vi "tagDB_setValue_Template.vi"(8 "Error In":errorcluster, 9 "value":variant, 10 "name":string, 11 "DB Ref":T1) -> (0 "Error Out":errorcluster, 1 "created?":bool, 3 "DB Ref(dup)":T1)   [LabVIEW 2014, in "TagDB(dev).lvlib"]
doc: "[Covers: REQ_TAGDB_TEMPLATE_SETVALUE]"
uses:
  tagDB_Def.ctl
  TagDB(dev).lvlib
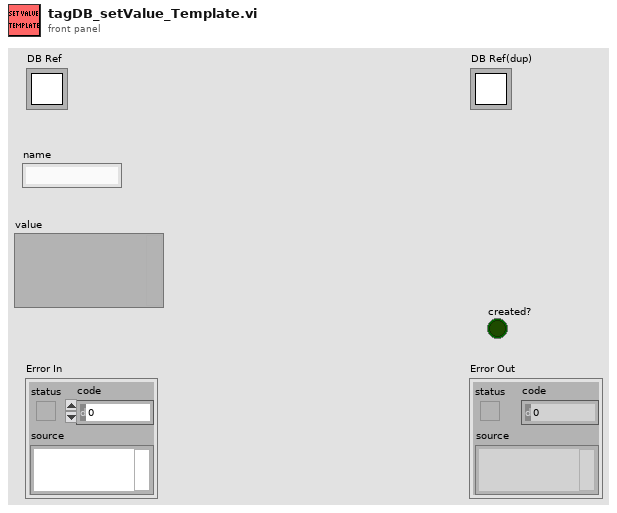
[diagram p1: front panel]
types:
  T1 = typedef "TagDB(dev).lvlib/tagDB_Def.ctl" = refnum<k1>
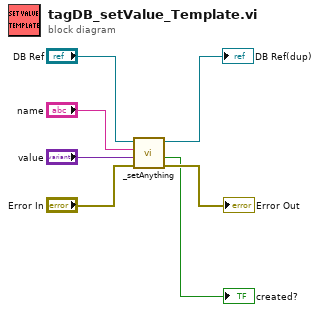
[diagram p0: block diagram]
diagram:
  n1 = call "_setAnything.vi"("Error In"="Error In", "value"="value", "name"="name", "DB Ref"="DB Ref") -> ("Error Out"=→"Error Out":errorcluster, "created?"=→"created?":bool, "DB Ref(dup)"=→"DB Ref(dup)":T1)  [unwired: 5 in]
